vi "Elapsed Time.vi"(7 "Start Time (ms)":u32, 11 "error in (no error)":errorcluster) -> (8 "MinSec string":string, 15 "error out":errorcluster)   [LabVIEW 2015]
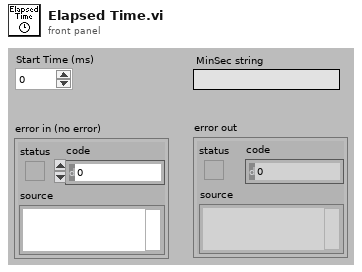
[diagram p1: front panel]
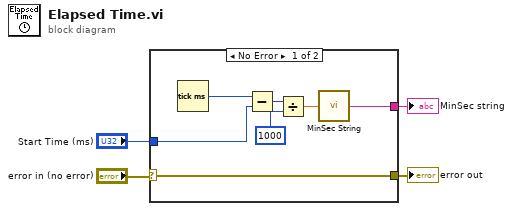
[diagram p0: block diagram]
diagram:
  n1 = case shown="No Error" "error in (no error)" {
    selector: "error in (no error)" -> [w11 w12]
    tunnel: [w11 w12] -> w3
    tunnel: "Start Time (ms)" -> [w9 _]
    tunnel: [w5 _] -> w1
    frame No Error {
      n2 = Tick Count (ms)() -> (millisecond timer value=w10:u32)
      n3 = Subtract(x=w10, y=w9) -> (x-y=w8:u32)
      n4 = Divide(x=w8, y=u32 1000) -> (x/y=w6:dbl)
      n5 = call "MinSec String.vi"("Seconds"=w6) -> ("MinSec string"=w5:string)
    }
    frame Error {
    }
  }
  "error out" <- w3
  "MinSec string" <- w1
